vi "WriteRegister.vi"(5 "Registers Info":map{T1, T2}(c390), 7 "Device Address":u8, 8 "error in (no error)":errorcluster, 9 "Register Name":T1=enum."Frame Rate", 10 "DATA":u8[](array[numeric]), 11 "II2COUSB":refnum<class "II2COUSB.lvclass">) -> (0 "error out":errorcluster)   [LabVIEW 2020, in "CameraI2COUSB.lvlib" / "CameraDemo.lvclass"]
uses:
  CameraDemo.lvclass
  CameraDemo.lvclass/CameraDemo.ctl
  I2CDriver/II2COUSB/II2COUSB/I2CFlags.ctl
  I2CDriver/II2COUSB/II2COUSB/II2COUSB.lvclass
  TypeDef/RegisterName.ctl
  TypeDef/RegisterInfo.ctl
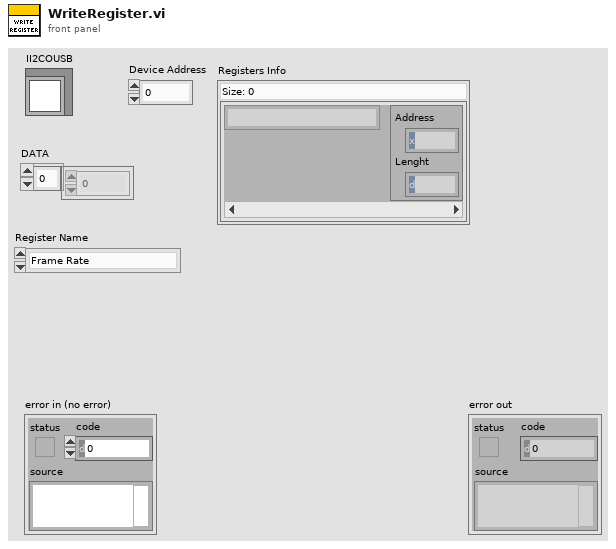
[diagram p1: front panel]
types:
  T1 = typedef "CameraI2COUSB.lvlib/CameraDemo.lvclass/RegisterName.ctl" = enum16{"Clock Rate", "Frame Rate", "Image Type", "Resolution", "Snap", "Start Streaming", "Stop Streaming"}
  T2 = typedef "CameraI2COUSB.lvlib/CameraDemo.lvclass/RegisterInfo.ctl" = cluster{"Address":u16, "Lenght":u32}
  T3 = typedef "II2COUSB.lvlib/II2COUSB.lvclass/I2CFlags.ctl" = u8
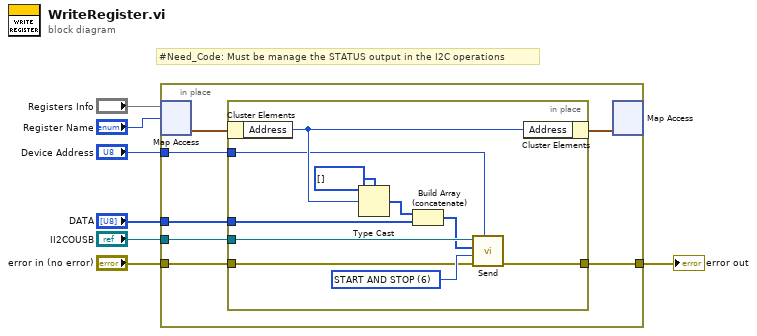
[diagram p0: block diagram]
diagram:
  # "#Need_Code: Must be manage the STATUS output in the I2C operations"
  n1 = in-place {
    in-place-border: "II2COUSB" -> [w13]
    in-place-border: "error in (no error)" -> [w12]
    in-place-border: [w8] -> w2
    in-place-border: "Device Address" -> [w11]
    in-place-border: "DATA" -> [w9]
    n2 = in-place-map #1("Registers Info", "Register Name") -> (w14:T2)  [unwired: 1 in, 1 out]
    n3 = in-place {
      in-place-border: w13 -> [w20]
      in-place-border: w12 -> [w21]
      in-place-border: w11 -> [w19]
      in-place-border: w9 -> [w17]
      in-place-border: [w15] -> w8
      w23 = T3 6 items=["None"=0, "START"=2, "REPEATED START"=3, "STOP"=4, "START AND STOP"=6] ("eI2Cflags")
      n4 = in-place-cluster #2(w14) -> ("Address"=w22:u16)
      n5 = Type Cast(type=u8[] [], x=w22) -> (*(type *) &x=w18:u8[])
      n6 = Build Array (concatenate)(w18, w17) -> (w16:u8[])
      n7 = call-dynamic "Send.vi"("Device Address"=w19, "error in (no error)"=w21, "eI2Cflags"=w23, "Buffer"=w16, "II2COUSB in"=w20) -> ("error out"=w15:errorcluster)  [unwired: 3 in, 3 out]
      n8 = in-place-cluster #2("Address"=w22) -> (w10:T2)
    }
    n9 = in-place-map #1(w10) -> ()  [unwired: 1 in, 3 out]
  }
  "error out" <- w2
